vi "Demo - Object Data.vi"() -> ()   [LabVIEW 2010]
uses:
  ListNode/ListNode.lvclass
  DoubleLinkedList/DoubleLinkedList.lvclass
  CustomeData/CustomeData.lvclass
panel:
  out "error out":errorcluster
  out "data":i32[](array[numeric])
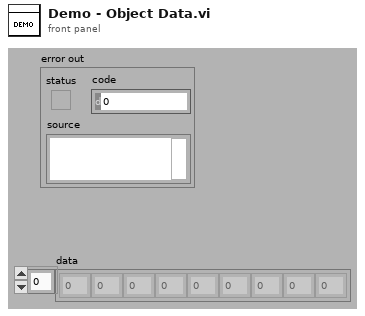
[diagram p1: front panel]
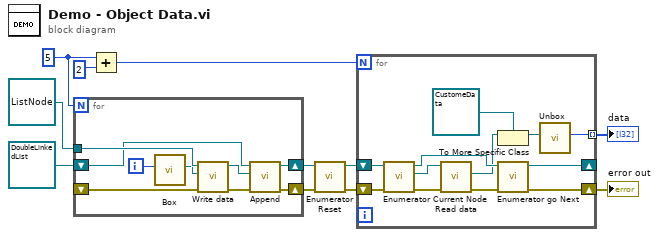
[diagram p0: block diagram]
diagram:
  w8 = 5
  n1 = for {
    N: w8 -> [_]
    tunnel: refnum<class "ListNode.lvclass"> refnum ("Node.lvclass") -> [w20]
    shift-right: [w12] -> w5
    shift-left: refnum<class "DoubleLinkedList.lvclass"> refnum ("List.lvclass") -> [w16]
    shift-right: [w13] -> w4
    shift-left: _ -> [w19]
    i -> [w18]
    n2 = call "Box.vi"("data"=w18) -> ("CustomeData out"=w17:refnum<class "CustomeData.lvclass">)  [unwired: 10 in]
    n3 = call-dynamic "Write data.vi"("error in (no error)"=w19, "data"=w17, "Node in"=w20) -> ("error out"=w14:errorcluster, "Node out"=w15:refnum<class "ListNode.lvclass">)  [unwired: 7 in]
    n4 = call-dynamic "Append.vi"("error in (no error)"=w14, "list node"=w15, "List in"=w16) -> ("error out"=w13:errorcluster, "List out"=w12:refnum<class "DoubleLinkedList.lvclass">)  [unwired: 7 in]
  }
  n5 = Add(x=w8, y=2) -> (x+y=w6:i32)
  n6 = call-dynamic "Enumerator Reset.vi"("error in (no error)"=w4, "List in"=w5) -> ("error out"=w3:errorcluster, "List out"=w2:refnum<class "DoubleLinkedList.lvclass">)  [unwired: 8 in]
  n7 = for {
    N: w6 -> [_]
    shift-right: [w32] -> _
    shift-left: w2 -> [w26]
    shift-right: [w31] -> w9
    shift-left: w3 -> [w25]
    tunnel: [w24] -> w1 mode=indexing
    n8 = call-dynamic "Enumerator Current Node.vi"("error in (no error)"=w25, "List in"=w26) -> ("error out"=w27:errorcluster, "Node"=w28:refnum<class "ListNode.lvclass">, "List out"=w29:refnum<class "DoubleLinkedList.lvclass">)  [unwired: 7 in]
    n9 = call-dynamic "Read data.vi"("error in (no error)"=w27, "Node in"=w28) -> ("error out"=w30:errorcluster, "data"=w22:refnum<class>)  [unwired: 7 in, 1 out]
    n10 = To More Specific Class(target class=refnum<class "CustomeData.lvclass"> refnum ("CustomeData.lvclass"), reference=w22) -> (specific class reference=w21:refnum<class "CustomeData.lvclass">)  [unwired: 1 in, 1 out]
    n11 = call-dynamic "Enumerator go Next.vi"("error in (no error)"=w30, "List in"=w29) -> ("error out"=w31:errorcluster, "List out"=w32:refnum<class "DoubleLinkedList.lvclass">)  [unwired: 8 in]
    n12 = call "Unbox.vi"("CustomeData in"=w21) -> ("data"=w24:i32)  [unwired: 10 in]
  }
  "data" <- w1
  "error out" <- w9
